vi "Read PS3 Camera.vi"() -> ()   [LabVIEW 2017]
uses:
  <vilib>/userdefined/High Color/IMAQdx.ctl
  <vilib>/vision/driver/NI_Vision_Acquisition_Software.lvlib
  <resource>/objmgr/imaqdx.rc
panel:
  out "Camera Information Array":T1(array[cluster]) {"BusType" format="%x"; "SerialNumberLow" format="%.0x"; "SerialNumberHigh" format="%.0x"}
  in  "Session In":T2
  out "The video mode that we set":u32
  in  "Set video mode to:":u32=159
  out "Default video mode of camera":u32
  out "Video Modes":T3(array[cluster])
  out "Error Out":errorcluster
  in  "Stop Button":bool
  out "Sony PS3 EYE camera":T4(plugin-control)
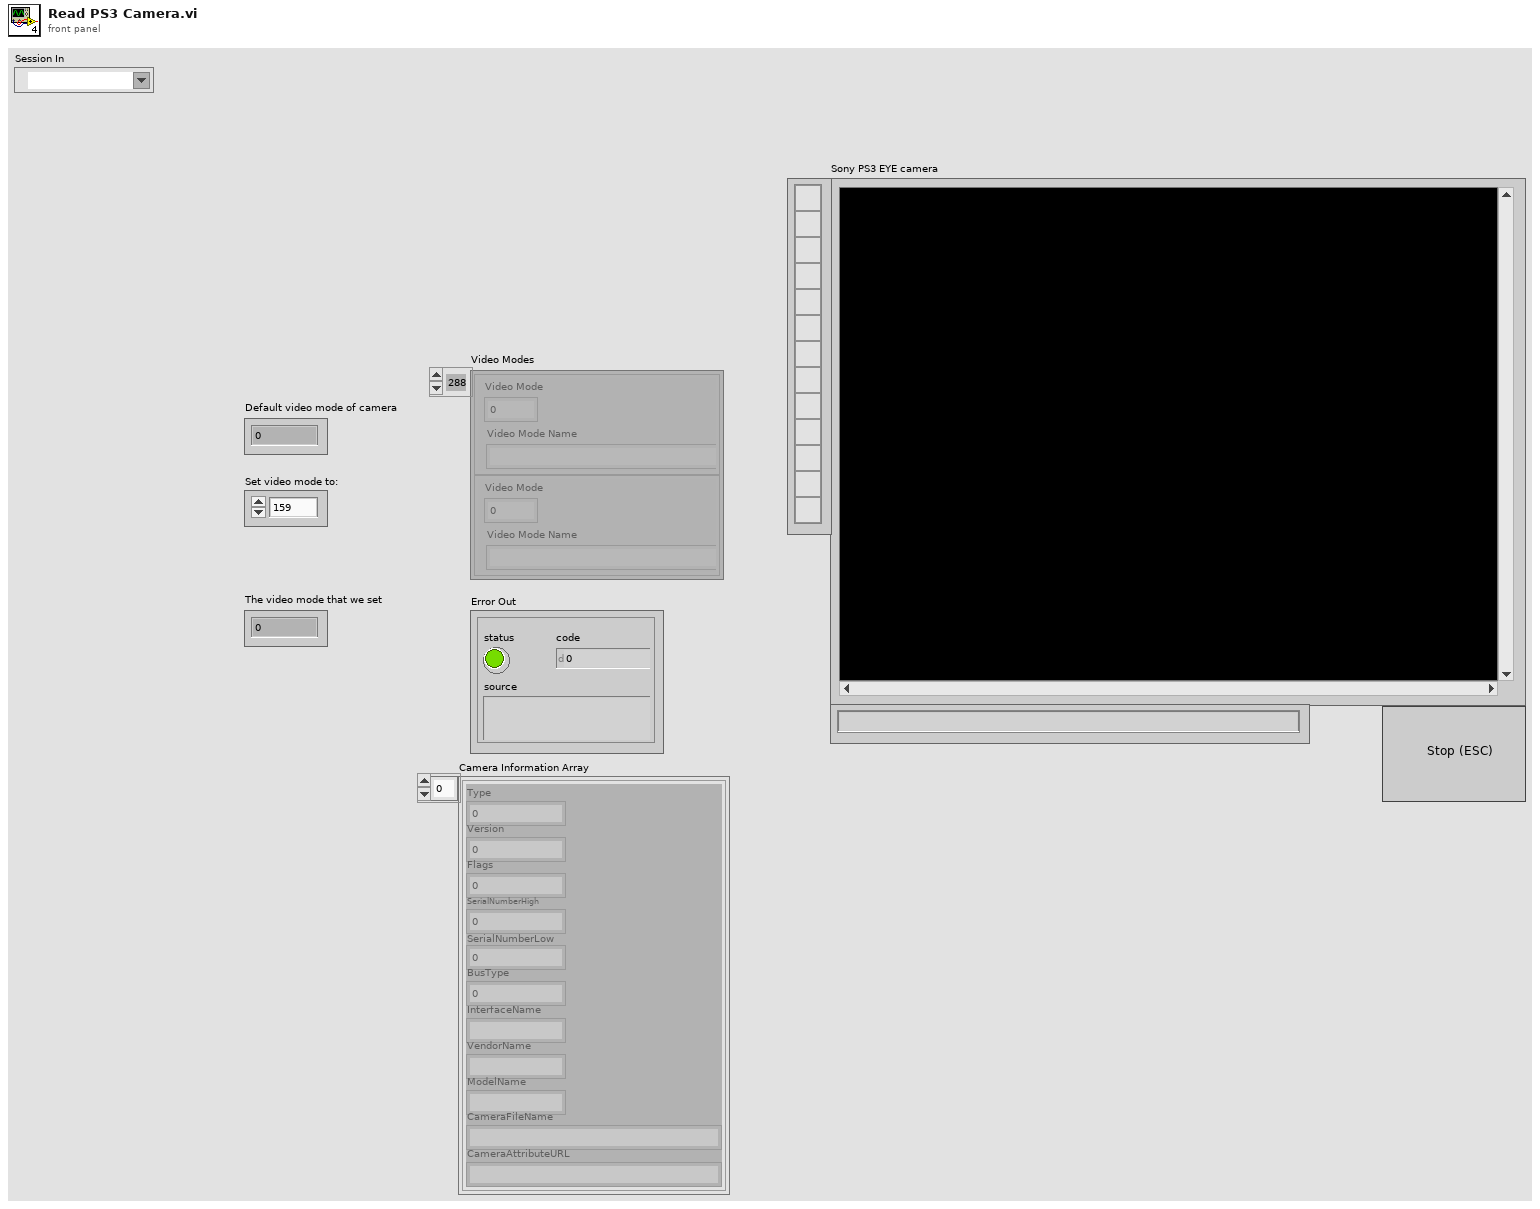
[diagram p1: front panel]
types:
  T1 = cluster{"Type":u32, "Version":u32, "Flags":u32, "SerialNumberHigh":u32, "SerialNumberLow":u32, "BusType":u32, "InterfaceName":string, "VendorName":string, "ModelName":string, "CameraFileName":string, "CameraAttributeURL":string}[]
  T2 = typedef "IMAQdx.ctl" = refnum<k21>
  T3 = cluster{"Video Mode":u32, "Video Mode Name":string}[]
  T4 = typedef "IMAQ Image.ctl" = refnum<image>
  T5 = typedef "Image Type" = u32
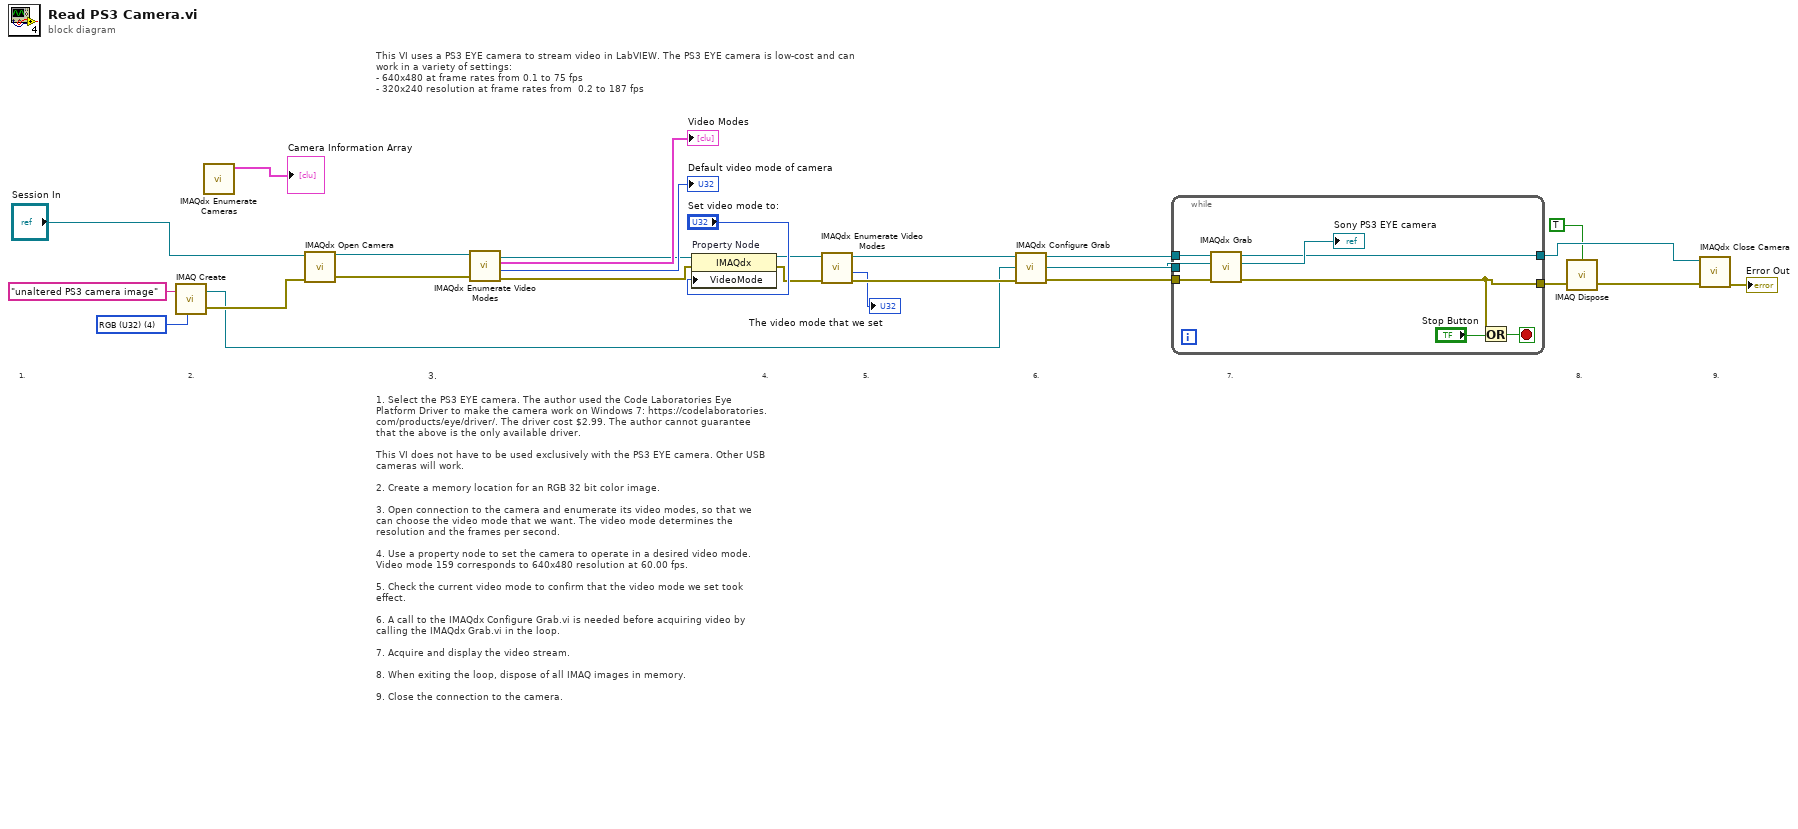
[diagram p0: block diagram]
diagram:
  w3 = T5 4 items=["Grayscale (U8)", "Grayscale (I16)", "Grayscale (SGL)", "Complex (CSG)", "RGB (U32)", "HSL (U32)", "RGB (U64)", "Grayscale (U16)"] ("Image Type")
  # "This VI uses a PS3 EYE camera to stream video in LabVIEW. The PS3 EYE camera is low-cost and can\nwork in a variety of settings:\n- 640x480 at frame rates from 0.1 to 75 fps \n- 320x240 resolution at frame rates from  0.2 to 187 fps"
  # "9."
  # "8."
  # "7."
  # "6."
  # "5."
  # "4."
  # "1."
  # "3."
  # "2."
  # "1. Select the PS3 EYE camera. The author used the Code Laboratories Eye Platform Driver to make the camera work on Windows 7: https://codelaboratories.com/products/eye/driver/. The driver cost $2.99. The author cannot guarantee that the above is the only available driver.\n\nThis VI does not have to be used exclusively with the PS3 EYE camera. Other USB cameras will work.\n\n2. Create a memory location for an RGB 32 bit color image.\n\n3. Open connection to the camera and enumerate its video modes, so that we can choose the video mode that we want. The video mode determines the resolution and the frames per second.\n\n4. Use a property node to set the camera to operate in a desired video mode. Video mode 159 corresponds to 640x480 resolution at 60.00 fps.\n\n5. Check the current video mode to confirm that the video mode we set took effect.\n\n6. A call to the IMAQdx Configure Grab.vi is needed before acquiring video by calling the IMAQdx Grab.vi in the loop.\n\n7. Acquire and display the video stream.\n\n8. When exiting the loop, dispose of all IMAQ images in memory.\n\n9. Close the connection to the camera."
  n1 = call "IMAQ Create"("Image Name"="unaltered PS3 camera image", "Image Type"=w3) -> ("New Image"=w5:T4, "error out"=w24:errorcluster)  [unwired: 3 in]
  n2 = call <vilib>:"IMAQdx Enumerate Cameras.vi"() -> ("Camera Information Array"=→"Camera Information Array":T1)  [unwired: 10 in, 1 out]
  n3 = call <vilib>:"IMAQdx Open Camera.vi"("error in"=w24, "Session In"="Session In") -> ("error out"=w16:errorcluster, "Session Out"=w17:T2)  [unwired: 8 in]
  n4 = call <vilib>:"IMAQdx Enumerate Video Modes.vi"("error in"=w16, "Session In"=w17) -> ("error out"=w12:errorcluster, "Current Mode"=→"Default video mode of camera":u32, "Video Modes"=→"Video Modes":T3, "Session Out"=w13:T2)  [unwired: 6 in]
  n5 = property on="Property Node" class="IMAQdx"(reference=w13, error in=w12, "VideoMode"="Set video mode to:") -> (reference out=w10:T2, error out=w9:errorcluster)
  n6 = call <vilib>:"IMAQdx Enumerate Video Modes.vi"("error in"=w9, "Session In"=w10) -> ("error out"=w8:errorcluster, "Current Mode"=→"The video mode that we set":u32, "Session Out"=w7:T2)  [unwired: 6 in, 1 out]
  n7 = call <vilib>:"IMAQdx Configure Grab.vi"("error in"=w8, "Session In"=w7) -> ("error out"=w22:errorcluster, "Session Out"=w23:T2)  [unwired: 8 in]
  n8 = while {
    tunnel: w22 -> [w33]
    tunnel: w23 -> [w32]
    tunnel: w5 -> [w31]
    tunnel: [w27] -> w20
    tunnel: [w26] -> w21
    stop <- w28 stop-if-true
    n9 = call <vilib>:"IMAQdx Grab.vi"("error in"=w33, "Image In"=w31, "Session In"=w32) -> ("error out"=w27:errorcluster, "Image Out"=→"Sony PS3 EYE camera":T4, "Session Out"=w26:T2)  [unwired: 5 in, 1 out]
    n10 = Or(x=w27, y="Stop Button") -> (x .or. y?=w28:bool)
  }
  n11 = call "IMAQ Dispose"("All Images? (No)"=TRUE, "error in (no error)"=w20) -> ("error out"=w19:errorcluster)  [unwired: 4 in]
  n12 = call <vilib>:"IMAQdx Close Camera.vi"("error in"=w19, "Session In"=w21) -> ("error out"=→"Error Out":errorcluster)  [unwired: 9 in]
